vi "Restore to default.vi"(8 "error in (no error)":errorcluster, 9 "NewVal":bool, 10 "Self Enqueuer":refnum<class "Message Enqueuer.lvclass">, 11 "ZenGage v3.0 UI in":refnum<class "ZenGage v3.0 UI.lvclass">) -> (0 "error out":errorcluster)   [LabVIEW 2015]
uses:
  ZenGage v3.0 UI.lvclass
  <vilib>/ActorFramework/Message Enqueuer/Message Enqueuer.lvclass
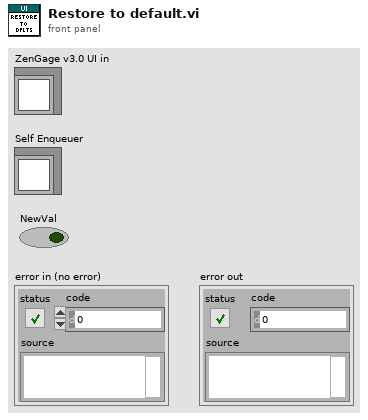
[diagram p1: front panel]
types:
  T1 = cluster{"Default JSON file path in":path, "Rack Controller Override JSON file path in":path, "Algo Parameters Override JSON file path in":path}
  T2 = cluster{"Default Override JSON":variant, "Rack Controller Override JSON":variant, "Algo Override JSON":variant}
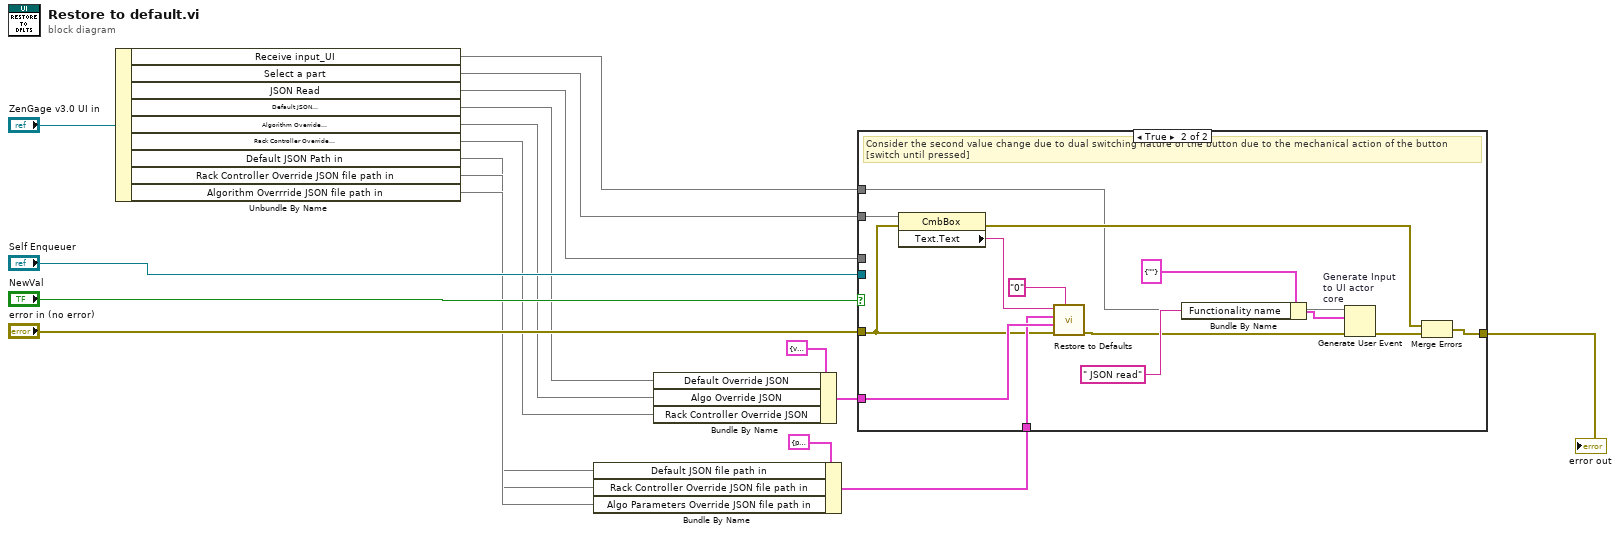
[diagram p0: block diagram]
diagram:
  n1 = Unbundle By Name("ZenGage v3.0 UI in") -> ("Receive input_UI"=w16, "Select a part"=w1, "JSON Read"=w2, "Default JSON \nVariant"=w4, "Algorithm Override\nJSON Variant"=w5, "Rack Controller Override\nJSON Variant"=w6, "Default JSON Path in"=w9, "Rack Controller Override JSON file path in"=w10, "Algorithm Overrride JSON file path in"=w11)
  n2 = Bundle By Name(cluster=T1 {"Default JSON file path in"=path "", "Rack Controller Override JSON file path in"=path "", "Algo Parameters Override JSON file path in"=path ""} ("JSON path cluster"), "Default JSON file path in"=w9, "Rack Controller Override JSON file path in"=w10, "Algo Parameters Override JSON file path in"=w11) -> (w12:T1)
  n3 = Bundle By Name(cluster=T2 {"Default Override JSON"=variant, "Rack Controller Override JSON"=variant, "Algo Override JSON"=variant} ("JSON Variant Clusters"), "Default Override JSON"=w4, "Algo Override JSON"=w5, "Rack Controller Override JSON"=w6) -> (w7:T2)
  n4 = case shown="True" "NewVal" {
    tunnel: w1 -> [_ w33]
    tunnel: w2 -> [_ _]
    tunnel: "error in (no error)" -> [w19 w28]
    tunnel: [w19 w26] -> w18
    tunnel: "Self Enqueuer" -> [_ _]
    tunnel: w7 -> [_ w30]
    tunnel: w12 -> [_ w29]
    tunnel: w16 -> [_ w20]
    frame False {
      # "Consider the first value change due to dual switching nature of the button due to the mechanical action of the button [switch until pressed]"
    }
    frame True {
      # "Consider the second value change due to dual switching nature of the button due to the mechanical action of the button [switch until pressed]"
      n5 = property class="CmbBox"(reference=w33, error in=w28) -> (error out=w27:errorcluster, "Text.Text"=w32:string)  [unwired: 1 out]
      n6 = call "Restore to Defaults.vi"("Rack Number"="0", "error in"=w28, "JSON Variant Clusters"=w30, "JSON path cluster"=w29, "Part Name in"=w32) -> ("error out"=w22:errorcluster)  [unwired: 6 in]
      n7 = Bundle By Name(cluster=cluster{"Functionality name":string} {"Functionality name"=""} ("event data"), "Functionality name"=" JSON read") -> (w24:cluster{"Functionality name":string})
      n8 = Generate User Event "Generate Input\nto UI actor\ncore"(user event=w20, event data cluster=w24, error in=w22) -> (error out=w21:errorcluster)  [unwired: 1 in, 1 out]
      n9 = Merge Errors(w27, w21) -> (w26:errorcluster)
    }
  }
  "error out" <- w18
